vi "Add Pulse Recorders.vi"(8 "error in (no error)":errorcluster, 9 "Auto launch":bool=TRUE, 10 "Module type":T1, 11 "Monitor-Pulse in":refnum<class "LabActor.lvclass">) -> (0 "error out":errorcluster, 1 "Actor names out":string[](array[string]), 2 "Recorders out":refnum<class "Pulse Recorder.lvclass">[](array[class]), 3 "Monitor-Pulse out":refnum<class "LabActor.lvclass">, 4 "Type IDs":i32[](array[numeric]))   [LabVIEW 2016, in "LabActor.lvclass"]
uses:
  LabActor.lvclass
  Pulse Recorders/Pulse Recorder/Pulse Recorder.lvclass
  C:/github/LabActor/Template Module/Template Module.lvclass
  C:/github/LabActor/Worker/Worker.lvclass
  Controllers/Application Controller/Module Types.ctl
  NHMFL_Core/Libraries/Instruments/Instrument Driver/Instrument Driver.lvclass/Instrument Driver.ctl
  Recorders/RP I-V/RP I-V.lvclass
  C:/github/LabActor/Pulse Recorders/Pulse Recorder/Pulse Recorder.lvclass
  Recorders/NI-Scope Lock-in/NI-Scope Lock-in.lvclass
  Template Module/Template Module.lvclass/Template Module.ctl
  NHMFL_Core/Libraries/Instruments/Instrument Driver/Read Type ID.vi
  Template Module/Write Name.vi
  NHMFL_Core/Libraries/Red Pitaya/Red Pitaya Digitizer/Red Pitaya Digitizer.lvclass
  C:/github/NHMFL_Core/Libraries/Instruments/Pulse Driver/Pulse Driver.lvclass
  NHMFL_Core/Libraries/Instruments/Pulse Driver/Pulse Driver.lvclass
  C:/github/NHMFL_Core/Libraries/Instruments/Instrument Driver/Instrument Driver.lvclass
  Pulse Recorders/Pulse Recorder/Write Pulse driver.vi
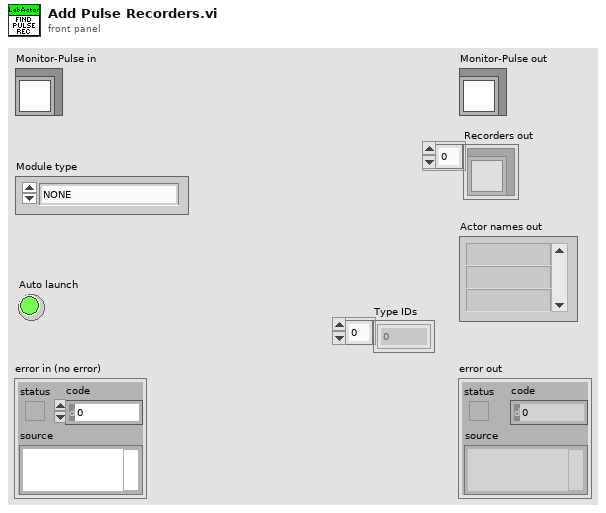
[diagram p1: front panel]
types:
  T1 = typedef "Module Types.ctl" = enum16{"NONE", "NI-DAQmx", "NI-Scope", "Red Pitaya Digitizer", "GaGe", "VISA Device", "Red Pitaya Lockin", "Monitor Controller", "Pulse Controller", "Integrate Pulse", "Lockin Processor", "File converter", "NHMFL Synthesizer", "Micron Hyperion", "Spectrum Recorder", "Resonance Detector", "TCP Communications", "Format Resonances"}
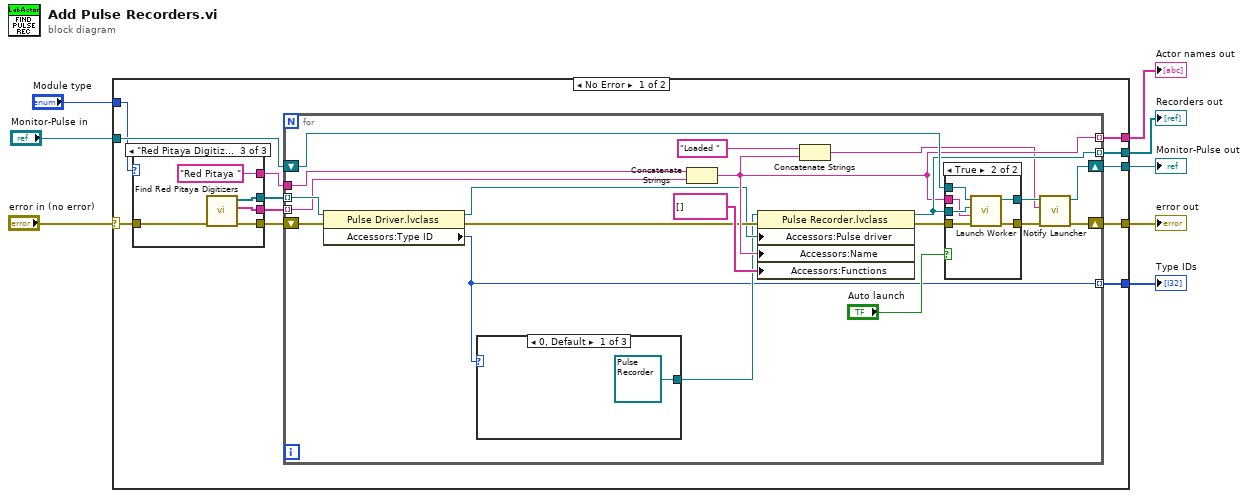
[diagram p0: block diagram]
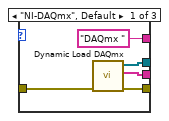
[diagram p2: hidden frame]
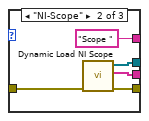
[diagram p3: hidden frame]
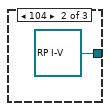
[diagram p4: hidden frame]
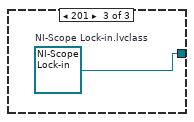
[diagram p5: hidden frame]
diagram:
  n1 = case shown="No Error" "error in (no error)" {
    selector: "error in (no error)" -> [w20 w68]
    tunnel: [w16 w68] -> w7
    tunnel: [w12 w67] -> w5
    tunnel: "Monitor-Pulse in" -> [w13 w67]
    tunnel: [w15 _] -> w4
    tunnel: [w14 _] -> w3
    tunnel: "Module type" -> [w11 _]
    tunnel: [w9 _] -> w1
    frame No Error {
      n2 = case shown="\"Red Pitaya Digitizer\"" w11 {
        tunnel: w20 -> [w25 w30 w35]
        tunnel: [w24 w27 w32] -> w19
        tunnel: [w23 w29 w31] -> w18
        tunnel: [w22 w28 w34] -> w17
        tunnel: ["DAQmx " "Scope " "Red Pitaya "] -> w10
        frame "NI-DAQmx", Default {
          n3 = call "Dynamic Load DAQmx.vi"("Error In"=w25) -> ("Error Out"=w23:errorcluster, "Device names"=w22:string[], "Digitizers out"=w24:refnum<class "Pulse Driver.lvclass">[])  [unwired: 8 in]
        }
        frame "NI-Scope" {
          n4 = call "Dynamic Load NI Scope.vi"("Error In"=w30) -> ("Error Out"=w29:errorcluster, "Device names"=w28:string[], "Digitizers out"=w27:refnum<class "Pulse Driver.lvclass">[])  [unwired: 8 in]
        }
        frame "Red Pitaya Digitizer" {
          n5 = call "Find Red Pitaya Digitizers.vi"("Error In"=w35) -> ("Error Out"=w31:errorcluster, "Device names"=w34:string[], "Digitizers out"=w32:refnum<class "Red Pitaya Digitizer.lvclass">[])  [unwired: 7 in, 1 out]
        }
      }
      n6 = for {
        tunnel: w19 -> [w40] mode=indexing
        shift-right: [w46] -> w16
        shift-left: w18 -> [w55]
        tunnel: w17 -> [w37] mode=indexing
        tunnel: [w53] -> w15 mode=indexing
        tunnel: [w44] -> w14 mode=indexing
        shift-right: [w48] -> w12
        shift-left: w13 -> [w54]
        tunnel: w10 -> [w50]
        tunnel: [w36] -> w9 mode=indexing
        n7 = property class="Pulse Driver.lvclass"(reference=w40, error in=w55) -> (reference out=w39:refnum<class "Pulse Driver.lvclass">, error out=w41:errorcluster, "Accessors:Type ID"=w36:i32)
        n8 = case shown="0, Default" w36 {
          tunnel: [refnum<class "Pulse Recorder.lvclass"> refnum ("Pulse Recorder.lvclass") refnum<class "RP I-V.lvclass"> refnum ("RP I-V.lvclass") w58] -> w38
          frame 0, Default {
          }
          frame 104 {
          }
          frame 201 {
            w58 = refnum<class "NI-Scope Lock-in.lvclass"> refnum  # NI-Scope Lock-in.lvclass
          }
        }
        n9 = Concatenate Strings(w50, w37) -> (w44:string)
        n10 = property class="Pulse Recorder.lvclass"(reference=w38, error in=w41, "Accessors:Pulse driver"=w39, "Accessors:Name"=w44, "Accessors:Functions"=string[] [] ("Functions")) -> (reference out=w53:refnum<class "Pulse Recorder.lvclass">, error out=w52:errorcluster)
        n11 = Concatenate Strings("Loaded " ("string"), w44) -> (w43:string)
        n12 = case shown="True" "Auto launch" {
          tunnel: w54 -> [w60 w66]
          tunnel: w53 -> [_ w65]
          tunnel: [w60 w64] -> w49
          tunnel: w52 -> [w59 w63]
          tunnel: [w59 w62] -> w47
          tunnel: w44 -> [_ w61]
          frame False {
          }
          frame True {
            n13 = call-dynamic "Launch Worker.vi"("error in (no error)"=w63, "Name"=w61, "Subordinate Object"=w65, "Application Controller in"=w66) -> ("error out"=w62:errorcluster, "Application Controller out"=w64:refnum<class "LabActor.lvclass">)  [unwired: 5 in, 1 out]
          }
        }
        n14 = call-dynamic "Notify Launcher.vi"("error in (no error)"=w47, "Notification"=w43, "Application Controller in"=w49) -> ("error out"=w46:errorcluster, "Application Controller out"=w48:refnum<class "LabActor.lvclass">)  [unwired: 7 in]
      }
    }
    frame Error {
    }
  }
  "error out" <- w7
  "Monitor-Pulse out" <- w5
  "Recorders out" <- w4
  "Actor names out" <- w3
  "Type IDs" <- w1
